vi "YAML Get Field Value Int.vi"(10 "field name":string, 11 "array of strings":string[][](array[string])) -> (3 "Numeric Control":i32)   [LabVIEW 2011]
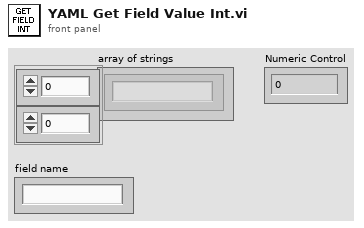
[diagram p1: front panel]
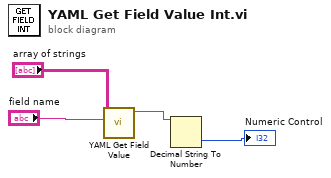
[diagram p0: block diagram]
diagram:
  n1 = call "YAML Get Field Value.vi"("field name"="field name", "array of strings"="array of strings") -> ("field value"=w2:string)  [unwired: 9 in]
  n2 = Decimal String To Number(string=w2) -> (number=→"Numeric Control":i32)  [unwired: 2 in, 1 out]
